vi "Configure Spot ENR.vi"(0 "VISA resource name":refnum<visa-resource-name>, 5 "Spot ENR Mode (0: ENR)":i32(ring) items=["ENR", "T-Hot"], 7 "ENR Spot Value (15.2 dB)":dbl=15.2 format="%^#_6g", 9 "ENR T-Hot Value (9892.8 K)":dbl=9892.8 format="%^#_6g", 11 "error in (no error)":errorcluster) -> (4 "VISA resource name out":refnum<visa-resource-name>, 15 "error out":errorcluster)   [LabVIEW 2014, in "Agilent ESA PSA Series.lvlib"]
doc: "Configures the spot ENR mode of the Noise Figure personality.\n\n<B>Note:</B> \n\nThis VI is only valid in Noise Figure personality. Use <B>Switch Personality</B> VI to switch to Noise Figure before calling this VI."
uses:
  Agilent ESA PSA Series.lvlib
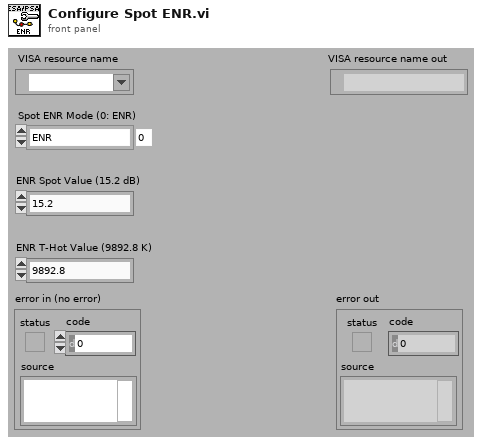
[diagram p1: front panel]
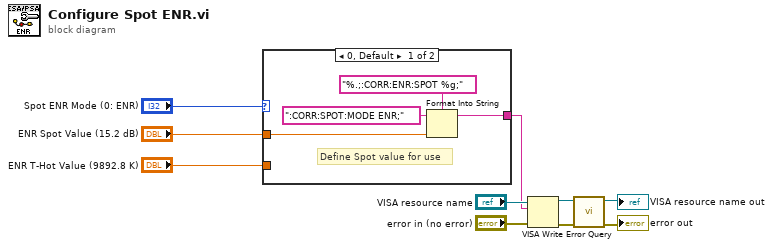
[diagram p0: block diagram]
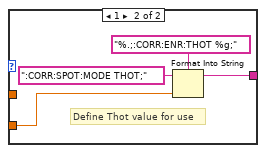
[diagram p2: hidden frame]
diagram:
  n1 = case shown="0, Default" "Spot ENR Mode (0: ENR)" {
    tunnel: "ENR Spot Value (15.2 dB)" -> [w14 _]
    tunnel: "ENR T-Hot Value (9892.8 K)" -> [_ w18]
    tunnel: [w11 w15] -> w1
    frame 0, Default {
      # "Define Spot value for use"
      n2 = Format Into String(format string="%.;:CORR:ENR:SPOT %g;", initial string=":CORR:SPOT:MODE ENR;", w14) -> (resulting string=w11:string)  [unwired: 1 in, 1 out]
    }
    frame 1 {
      # "Define Thot value for use"
      n3 = Format Into String(format string="%.;:CORR:ENR:THOT %g;", initial string=":CORR:SPOT:MODE THOT;", w18) -> (resulting string=w15:string)  [unwired: 1 in, 1 out]
    }
  }
  n4 = VISA Write(VISA resource name="VISA resource name", write buffer=w1, error in (no error)="error in (no error)") -> (VISA resource name out=w8:refnum<visa-resource-name>, error out=w7:errorcluster)  [unwired: 1 out]
  n5 = call "Error Query.vi"("error in (no error)"=w7, "VISA resource name"=w8) -> ("error out"=→"error out":errorcluster, "VISA resource name out"=→"VISA resource name out":refnum<visa-resource-name>)  [unwired: 6 in, 2 out]
